vi "Update Water Level.vi"(8 "error in (no error)":cluster{"状态":bool, "代码":i32, "源":string} caption="错误输入（无错误）", 10 "水位":dbl, 11 "蒸发冷却器的控制器输入":refnum<class "Evaporative Cooler Controller.lvclass">) -> (0 "error out":cluster{"状态":bool, "代码":i32, "源":string} caption="错误输出", 3 "蒸发冷却器的控制器输出":refnum<class "Evaporative Cooler Controller.lvclass">)   [LabVIEW 2013, in "Evaporative Cooler Controller.lvlib" / "Evaporative Cooler Controller.lvclass"]
doc: "子类中必须对该方法进行重写以显示水槽中水深的新状态或更新记录文件。"
uses:
  Evaporative Cooler Controller.lvclass
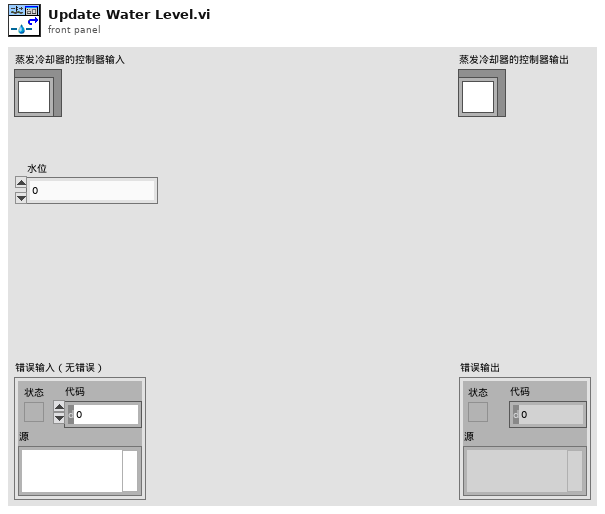
[diagram p1: front panel]
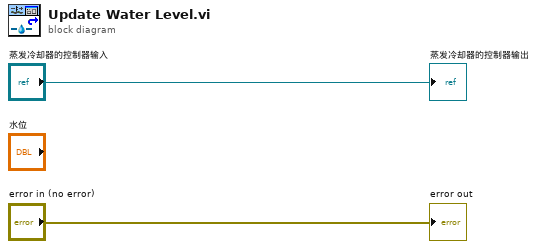
[diagram p0: block diagram]
diagram:
  "error out" <- "error in (no error)"
  "蒸发冷却器的控制器输出" <- "蒸发冷却器的控制器输入"
